vi "Prepare SQL Statement for Cluster.vi"(8 "error in (no error)":errorcluster, 9 "Columns":T1[](array[typedef])=[{"Include"=TRUE, "Name"="Position", "SQLite3 type"=enum."SQLITE_FLOAT"}, {"Include"=TRUE, "Name"="Event Type", "SQLite3 type"=enum."SQLITE_INTEGER"}, {"Include"=TRUE, "Name"="Area", "SQLite3 type"=enum."SQLITE_INTEGER"}, {"Include"=TRUE, "Name"="Channels", "SQLite3 type"=enum."SQLITE_INTEGER"}, {"Include"=TRUE, "Name"="Start position", "SQLite3 type"=enum."SQLITE_INTEGER"}, {"Include"=TRUE, "Name"="End  position", "SQLite3 type"=enum."SQLITE_INTEGER"}, {"Include"=TRUE, "Name"="Name", "SQLite3 type"=enum."SQLITE3_TEXT"}, {"Include"=TRUE, "Name"="Offset", "SQLite3 type"=enum."SQLITE_INTEGER"}, {"Include"=TRUE, "Name"="Length", "SQLite3 type"=enum."SQLITE_INTEGER"}, {"Include"=TRUE, "Name"="Action marker", "SQLite3 type"=enum."SQLITE3_TEXT"}, {"Include"=TRUE, "Name"="Event", "SQLite3 type"=enum."SQLITE_INTEGER"}, {"Include"=TRUE, "Name"="# Defects", "SQLite3 type"=enum."SQLITE_INTEGER"}, {"Include"=TRUE, "Name"="jpg Image", "SQLite3 type"=enum."SQLITE3_TEXT"}, {"Include"=TRUE, "Name"="chan maxs", "SQLite3 type"=enum."SQLITE_INTEGER"}, {"Include"=TRUE, "Name"="chan mins", "SQLite3 type"=enum."SQLITE_INTEGER"}, {"Include"=TRUE, "Name"="TimeStamp", "SQLite3 type"=enum."SQLITE_INTEGER"}, {"Include"=TRUE, "Name"="Readings", "SQLite3 type"=enum."SQLITE3_TEXT"}, {"Include"=TRUE, "Name"="ID", "SQLite3 type"=enum."SQLITE_INTEGER"}, {"Include"=TRUE, "Name"="New", "SQLite3 type"=enum."SQLITE_INTEGER"}, {"Include"=TRUE, "Name"="Hires Track", "SQLite3 type"=enum."SQLITE_INTEGER"}, {"Include"=TRUE, "Name"="2D overlay", "SQLite3 type"=enum."SQLITE_INTEGER"}, {"Include"=TRUE, "Name"="update", "SQLite3 type"=enum."SQLITE_INTEGER"}, {"Include"=TRUE, "Name"="Field #", "SQLite3 type"=enum."SQLITE_INTEGER"}, {"Include"=TRUE, "Name"="Events Class", "SQLite3 type"=enum."SQLITE_INTEGER"}, {"Include"=TRUE, "Name"="Sync", "SQLite3 type"=enum."SQLITE_INTEGER"}, {"Include"=TRUE, "Name"="Insert Offset", "SQLite3 type"=enum."SQLITE_INTEGER"}, {"Include"=TRUE, "Name"="Next trend", "SQLite3 type"=enum."SQLITE_INTEGER"}, {"Include"=TRUE, "Name"="Speed", "SQLite3 type"=enum."SQLITE_INTEGER"}], 10 "Table":string, 11 "SQLite Connection in":refnum<class "Connection.lvclass">) -> (0 "error out":errorcluster, 2 "SQL Statement":refnum<class "SQL Statement.lvclass">, 3 "SQLite Connection out":refnum<class "Connection.lvclass">, 5 "concatenated string":string)   [LabVIEW 2017]
doc: "Adds a new album to the database."
uses:
  <vilib>/drjdpowell/SQLite Library/SQL Connection/Connection.lvclass
  Common64/Database/SQ Lite/SQ Lite Cluster Action.ctl
  <vilib>/drjdpowell/SQLite Library/SQL Statement/SQL Statement.lvclass
  Beltwatch/BeltWatch 4-2-2-5/Database/Beltwatch SQLite.lvlib
panel:
  in  "ReadingsCols":T1[](array[typedef])=[{"Include"=TRUE, "Name"="Reading #", "SQLite3 type"=enum."SQLITE_INTEGER"}, {"Include"=TRUE, "Name"="Readings", "SQLite3 type"=enum."SQLITE3_TEXT"}, {"Include"=TRUE, "Name"="Reading Name", "SQLite3 type"=enum."SQLITE3_TEXT"}, {"Include"=TRUE, "Name"="TypeVal", "SQLite3 type"=enum."SQLITE_INTEGER"}, {"Include"=TRUE, "Name"="Alarm priority", "SQLite3 type"=enum."SQLITE_INTEGER"}, {"Include"=FALSE, "Name"="Display precision", "SQLite3 type"=enum."undefined type (0)"}, {"Include"=TRUE, "Name"="TypeStr", "SQLite3 type"=enum."SQLITE3_TEXT"}, {"Include"=TRUE, "Name"="AlarmPriorityStr", "SQLite3 type"=enum."SQLITE3_TEXT"}]
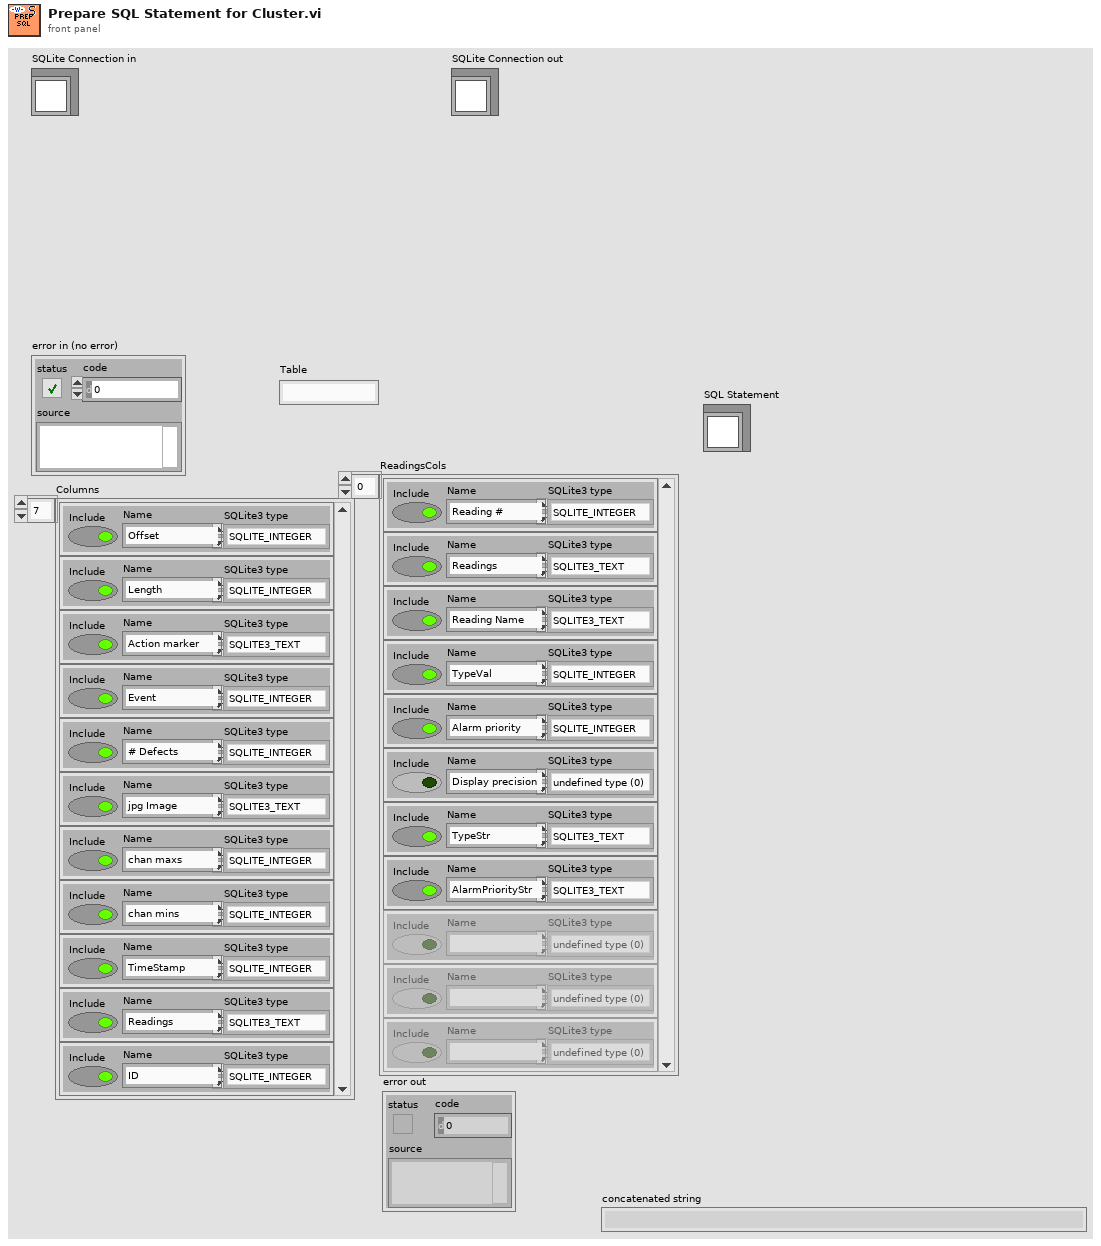
[diagram p1: front panel]
types:
  T1 = typedef "Beltwatch SQLite.lvlib/SQ Lite Cluster Action.ctl" = cluster{"Include":bool, "Name":string, "SQLite3 type":enum32{"undefined type (0)", "SQLITE_INTEGER", "SQLITE_FLOAT", "SQLITE3_TEXT", "SQLITE_BLOB", "SQLITE_NULL", "undefined type"}}
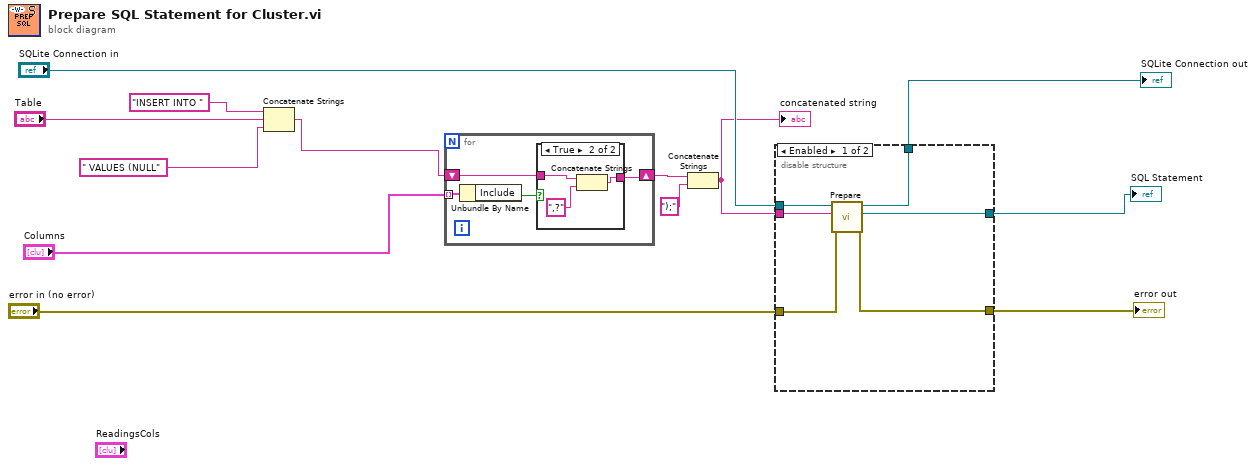
[diagram p0: block diagram]
diagram:
  n1 = Concatenate Strings("INSERT INTO ", "Table", " VALUES (NULL") -> (w2:string)
  n2 = for {
    tunnel: "Columns" -> [w17] mode=indexing
    shift-right: [w14] -> w9
    shift-left: w2 -> [w15]
    n3 = Unbundle By Name(w17) -> ("Include"=w16:bool)
    n4 = case shown="True" w16 {
      tunnel: w15 -> [w18 w20]
      tunnel: [w18 w21] -> w14
      frame False {
      }
      frame True {
        n5 = Concatenate Strings(w20, ",?" ("string")) -> (w21:string)
      }
    }
  }
  n6 = Concatenate Strings(w9, ");" ("string")) -> (w7:string)
  "concatenated string" <- w7
  n7 = disable-structure shown="Enabled" {
    disable-tunnel: "SQLite Connection in" -> [w27 _]
    disable-tunnel: "error in (no error)" -> [w26 _]
    disable-tunnel: [w25 _] -> w11
    disable-tunnel: w7 -> [w24 _]
    disable-tunnel: [w23 _] -> w6
    disable-tunnel: [w22 _] -> w1
    frame Enabled {
      n8 = call <vilib>:"Prepare.vi"("error in (no error)"=w26, "SQL"=w24, "SQLite Connection in"=w27) -> ("error out"=w23:errorcluster, "SQL Statement"=w22:refnum<class "SQL Statement.lvclass">, "SQLite Connection"=w25:refnum<class "Connection.lvclass">)  [unwired: 4 in, 2 out]
    }
    frame Disabled {
    }
  }
  "SQLite Connection out" <- w11
  "error out" <- w6
  "SQL Statement" <- w1
